vi "Create and Open New Track.vi"(8 "Error In":errorcluster, 10 "Samples Per Channel":i32, 11 "Track Name":string) -> (0 "Error Out":errorcluster, 3 "Track (File) References":T1)   [LabVIEW 2014]
doc: "Create 4 new audio files based off the given file name. Each file is formatted with 1 Track each containing Left and Right channels. If a set of tracks with the same file name requested already exist, the files will be replaced. This VI returns a reference to each track file."
uses:
  Controls/Track (File) References.ctl
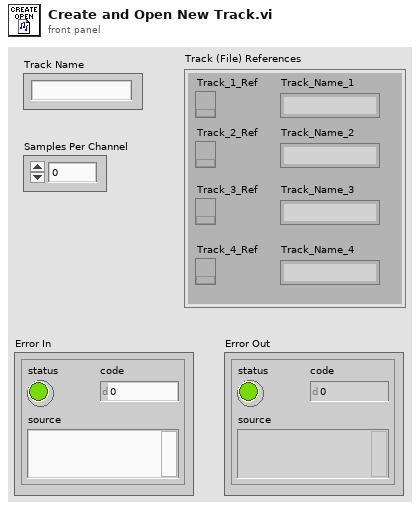
[diagram p1: front panel]
types:
  T1 = typedef "Track (File) References.ctl" = cluster{"Track_1_Ref":refnum<k34>, "Track_2_Ref":refnum<k34>, "Track_3_Ref":refnum<k34>, "Track_4_Ref":refnum<k34>, "Track_Name_1":string, "Track_Name_2":string, "Track_Name_3":string, "Track_Name_4":string}
  T2 = typedef "Track File Names.ctl" = cluster{"Track_1":string, "Track_2":string, "Track_3":string, "Track_4":string}
  T3 = cluster{"Track_1_Path":path, "Track_2_Path":path, "Track_3_Path":path, "Track_4_Path":path}
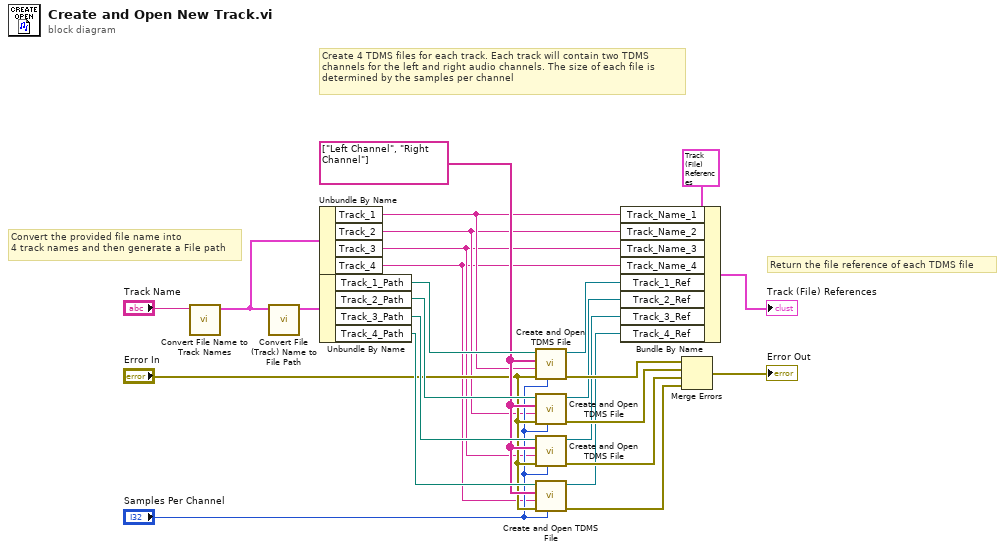
[diagram p0: block diagram]
diagram:
  w15 = string[] ["Left Channel", "Right Channel"] ("channel name(s)")
  # "Return the file reference of each TDMS file"
  # "Create 4 TDMS files for each track. Each track will contain two TDMS \nchannels for the left and right audio channels. The size of each file is \ndetermined by the samples per channel"
  # "Convert the provided file name into \n4 track names and then generate a File path"
  n1 = call "Convert File Name to Track Names.vi"("File Name"="Track Name") -> ("Track Names"=w22:T2)  [unwired: 10 in]
  n2 = call "Convert File (Track) Name to File Path.vi"("Track Names"=w22) -> ("Track File Paths"=w24:T3)  [unwired: 10 in]
  n3 = Unbundle By Name(w22) -> ("Track_1"=w4:string, "Track_2"=w3:string, "Track_3"=w2:string, "Track_4"=w1:string)
  n4 = Unbundle By Name(w24) -> ("Track_1_Path"=w23:path, "Track_2_Path"=w18:path, "Track_3_Path"=w17:path, "Track_4_Path"=w16:path)
  n5 = call "Create and Open TDMS File.vi"("Samples Per Channel"="Samples Per Channel", "Error In"="Error In", "TDMS Group Name"=w4, "TDMS Channel Name"=w15, "TDMS File Path"=w23) -> ("Error Out"=w21:errorcluster, "TDMS File Ref Out"=w19:refnum<k34>)  [unwired: 5 in]
  n6 = call "Create and Open TDMS File.vi"("Samples Per Channel"="Samples Per Channel", "Error In"="Error In", "TDMS Group Name"=w3, "TDMS Channel Name"=w15, "TDMS File Path"=w18) -> ("Error Out"=w10:errorcluster, "TDMS File Ref Out"=w8:refnum<k34>)  [unwired: 5 in]
  n7 = call "Create and Open TDMS File.vi"("Samples Per Channel"="Samples Per Channel", "Error In"="Error In", "TDMS Group Name"=w2, "TDMS Channel Name"=w15, "TDMS File Path"=w17) -> ("Error Out"=w9:errorcluster, "TDMS File Ref Out"=w7:refnum<k34>)  [unwired: 5 in]
  n8 = call "Create and Open TDMS File.vi"("Samples Per Channel"="Samples Per Channel", "Error In"="Error In", "TDMS Group Name"=w1, "TDMS Channel Name"=w15, "TDMS File Path"=w16) -> ("Error Out"=w5:errorcluster, "TDMS File Ref Out"=w6:refnum<k34>)  [unwired: 5 in]
  n9 = Bundle By Name(cluster=T1 {"Track_1_Ref"=refnum, "Track_2_Ref"=refnum, "Track_3_Ref"=refnum, "Track_4_Ref"=refnum, "Track_Name_1"="", "Track_Name_2"="", "Track_Name_3"="", "Track_Name_4"=""} ("Track (File) Refereces"), "Track_Name_1"=w4, "Track_Name_2"=w3, "Track_Name_3"=w2, "Track_Name_4"=w1, "Track_1_Ref"=w19, "Track_2_Ref"=w8, "Track_3_Ref"=w7, "Track_4_Ref"=w6) -> (→"Track (File) References":T1)
  n10 = Merge Errors(w21, w10, w9, w5) -> (→"Error Out":errorcluster)
